vi "CS-4 Set Ranges.vi"(2 "error in (no error)":errorcluster, 3 "range 1":dbl format="%.2f", 4 "range 0":dbl format="%.2f", 5 "VISA session":refnum<visa-resource-name>) -> (0 "error out":errorcluster, 1 "dup VISA session":refnum<visa-resource-name>)   [LabVIEW 2016]
doc: "CS-4 Set Ranges.vi sets the sweep ranges used for different sweep rates."
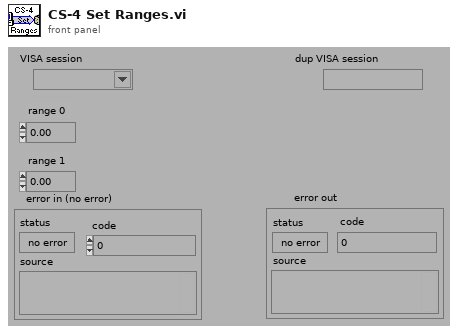
[diagram p1: front panel]
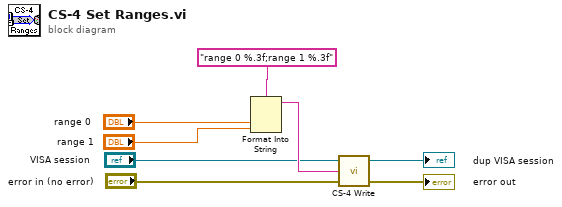
[diagram p0: block diagram]
diagram:
  n1 = Format Into String(format string="range 0 %.3f;range 1 %.3f", "range 0", "range 1") -> (resulting string=w6:string)  [unwired: 2 in, 1 out]
  n2 = call "CS-4 Write.vi"("error in (no error)"="error in (no error)", "write buffer (\"\")"=w6, "VISA session"="VISA session") -> ("error out"=→"error out":errorcluster, "dup VISA session"=→"dup VISA session":refnum<visa-resource-name>)  [unwired: 1 out]
